vi "坐标旋转.vi"(9 "旋转角度(单位°)":dbl, 11 "dtx,dty In":cluster{"X":dbl, "Y":dbl}) -> (3 "dtx,dty Out":cluster{"X":dbl, "Y":dbl})   [LabVIEW 2014]
uses:
  <vilib>/vision/NI_Vision_Development_Module.lvlib
panel:
  out "Angles (deg)":sgl[](array[numeric]) format="%.2f"
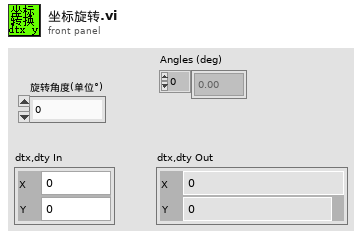
[diagram p1: front panel]
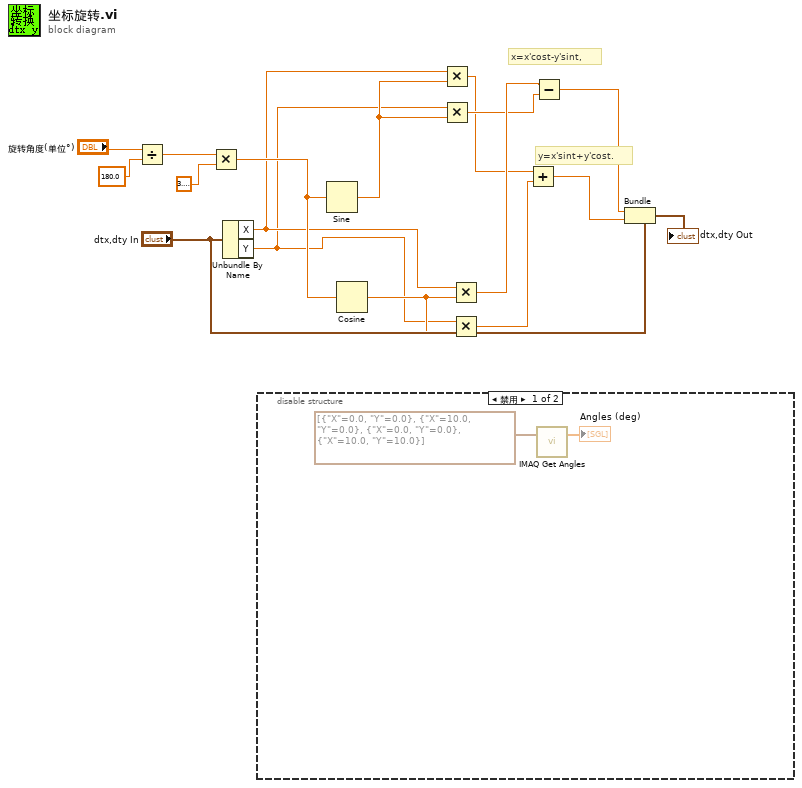
[diagram p0: block diagram]
diagram:
  # "y=x'sint+y'cost."
  # "x=x'cost-y'sint,"
  n1 = Divide(x="旋转角度(单位°)", y=180.0) -> (x/y=w13:dbl)
  n2 = Multiply(x=w13, y=3.141592653589793) -> (x*y=w11:dbl)
  n3 = Unbundle By Name("dtx,dty In") -> ("X"=w9:dbl, "Y"=w7:dbl)
  n4 = disable-structure shown="禁用" {
    frame Disabled {
      n5 = call "IMAQ Get Angles"("Points"=cluster{"X":sgl, "Y":sgl}[] [{"X"=0.0, "Y"=0.0}, {"X"=10.0, "Y"=0.0}, {"X"=0.0, "Y"=0.0}, {"X"=10.0, "Y"=10.0}]) -> ("Angles (deg)"=→"Angles (deg)":sgl[])  [unwired: 4 in, 2 out]
    }
    frame Enabled {
    }
  }
  n6 = Sine(x=w11) -> (sin(x)=w10:dbl)
  n7 = Cosine(x=w11) -> (cos(x)=w8:dbl)
  n8 = Multiply(x=w9, y=w10) -> (x*y=w4:dbl)
  n9 = Multiply(x=w7, y=w10) -> (x*y=w5:dbl)
  n10 = Multiply(x=w9, y=w8) -> (x*y=w6:dbl)
  n11 = Multiply(x=w7, y=w8) -> (x*y=w3:dbl)
  n12 = Add(x=w4, y=w3) -> (x+y=w1:dbl)
  n13 = Subtract(x=w6, y=w5) -> (x-y=w2:dbl)
  n14 = Bundle(cluster="dtx,dty In", "X"=w2, "Y"=w1) -> (→"dtx,dty Out":cluster{"X":dbl, "Y":dbl})
